vi "ROI entry-Check ROI Z range.vi"(10 "[AOL Z  (um)] previous":dbl[](array[numeric]), 11 "[AOL Z  (um)] Latest":dbl[](array[numeric])) -> (3 "All Z values in range ?":bool)   [LabVIEW 2020]
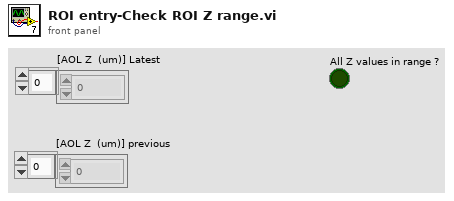
[diagram p1: front panel]
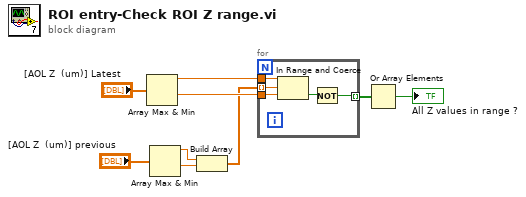
[diagram p0: block diagram]
diagram:
  n1 = Array Max & Min(array="[AOL Z  (um)] Latest") -> (max value=w9:dbl, min value=w8:dbl)  [unwired: 2 out]
  n2 = Array Max & Min(array="[AOL Z  (um)] previous") -> (max value=w7:dbl, min value=w6:dbl)  [unwired: 2 out]
  n3 = Build Array(w7, w6) -> (w5:dbl[])
  n4 = for {
    tunnel: w9 -> [w14]
    tunnel: w8 -> [w13]
    tunnel: w5 -> [w12] mode=indexing
    tunnel: [w10] -> w2 mode=indexing
    n5 = In Range and Coerce(upper limit=w14, x=w12, lower limit=w13) -> (In Range?=w11:bool)  [unwired: 1 out]
    n6 = Not(x=w11) -> (.not. x?=w10:bool)
  }
  n7 = Or Array Elements(Boolean array=w2) -> (logical OR=→"All Z values in range ?":bool)
